vi "Test_Class Load.vi"() -> ()   [LabVIEW 2020]
uses:
  ClassLoader.lvlib
panel:
  out "Loaded Class":refnum<class>
  out "Success?":bool
  out "error out":errorcluster
  in  "error in (no error)":errorcluster
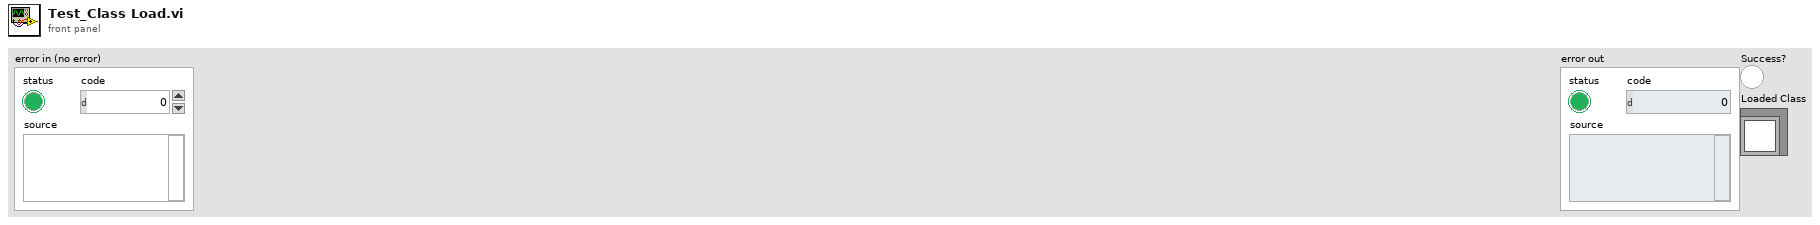
[diagram p1: front panel]
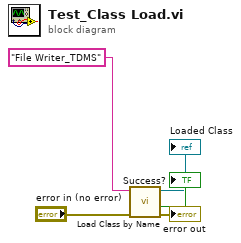
[diagram p0: block diagram]
diagram:
  n1 = call "Load Class by Name.vi"("error in (no error)"="error in (no error)", "Class Name"="File Writer_TDMS") -> ("error out"=→"error out":errorcluster, "Success?"=→"Success?":bool, "Loaded Class"=→"Loaded Class":refnum<class>)  [unwired: 7 in]
